vi "Uniform White Noise PtByPt.vi"(1 "initialize":bool, 2 "seed":i32=-1, 3 "amplitude":dbl=1.0 format="%0.2f") -> (0 "uniform white noise":dbl format="%0.2f")   [LabVIEW 2020, in "NI_PtbyPt.lvlib"]
doc: "Generates a uniformly distributed, pseudorandom pattern whose values are in the range [-a:a], where a is the absolute value of <B>amplitude</B>."
uses:
  NI_PtbyPt.lvlib
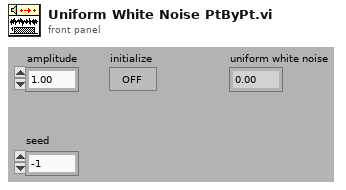
[diagram p1: front panel]
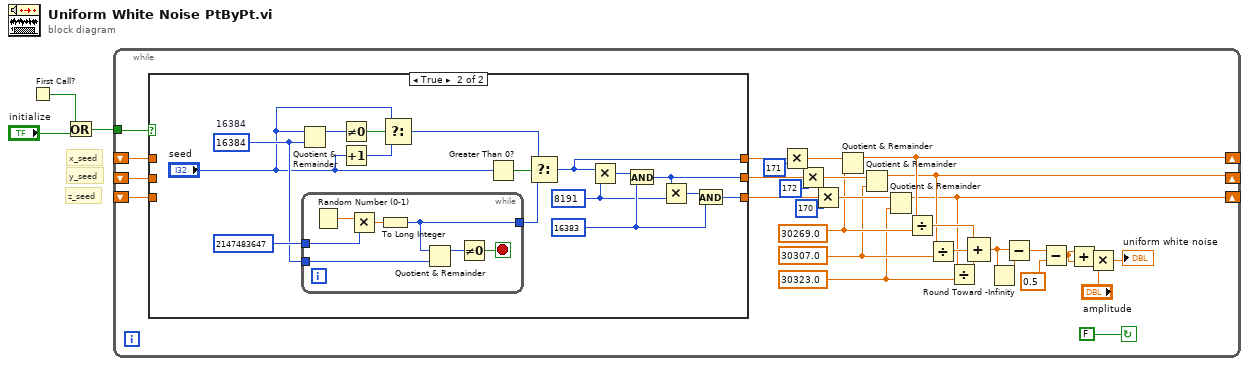
[diagram p0: block diagram]
diagram:
  # "z_seed"
  # "y_seed"
  # "x_seed"
  n1 = First Call?() -> (First Call?: T/F=w2:bool)
  n2 = Or(x=w2, y="initialize") -> (x .or. y?=w1:bool)
  n3 = while {
    tunnel: w1 -> [w10]
    shift-left: _ -> [w31]
    shift-right: [w12] -> _
    shift-left: _ -> [w32]
    shift-right: [w14] -> _
    shift-left: _ -> [w33]
    shift-right: [w16] -> _
    stop <- FALSE continue-if-true
    w11 = 30323.0
    w13 = 30307.0
    w15 = 30269.0
    n4 = case shown="True" w10 {
      tunnel: w33 -> [w37 _]
      tunnel: w32 -> [w36 _]
      tunnel: w31 -> [w35 _]
      tunnel: [w37 w38] -> w30
      tunnel: [w35 w53] -> w29
      tunnel: [w36 w52] -> w28
      frame False {
      }
      frame True {
        w46 = 16384  # 16384
        w50 = 16383
        w48 = 8191 ("y")
        n5 = Quotient & Remainder(x="seed", y=w46) -> (x-y*floor(x/y)=w41:i32)  [unwired: 1 out]
        n6 = while {
          tunnel: [w58] -> w45
          tunnel: w46 -> [w57]
          tunnel: 2147483647 ("x") -> [w54]
          stop <- w55 stop-if-true
          n7 = Random Number (0-1)() -> (number: 0 to 1=w59:dbl)
          n8 = Multiply(x=w59, y=w54) -> (x*y=w60:dbl)
          n9 = To Long Integer(number=w60) -> (32bit integer=w58:i32)
          n10 = Quotient & Remainder(x=w58, y=w57) -> (x-y*floor(x/y)=w56:i32)  [unwired: 1 out]
          n11 = Not Equal To 0?(x=w56) -> (x != 0?=w55:bool)
        }
        n12 = Not Equal To 0?(x=w41) -> (x != 0?=w42:bool)
        n13 = Increment(x="seed") -> (x+1=w43:i32)
        n14 = Select(t="seed", s=w42, f=w43) -> (s? t:f=w44:i32)
        n15 = Greater Than 0?(x="seed") -> (x > 0?=w40:bool)
        n16 = Select(t=w44, s=w40, f=w45) -> (s? t:f=w38:i32)
        n17 = Multiply(x=w38, y=w48) -> (x*y=w51:i32)
        n18 = And(x=w51, y=w50) -> (x .and. y?=w52:i32)
        n19 = Multiply(x=w52, y=w48) -> (x*y=w49:i32)
        n20 = And(x=w49, y=w50) -> (x .and. y?=w53:i32)
      }
    }
    n21 = Multiply(x=w30, y=171) -> (x*y=w17:dbl)
    n22 = Multiply(x=w28, y=172) -> (x*y=w25:dbl)
    n23 = Multiply(x=w29, y=170) -> (x*y=w24:dbl)
    n24 = Quotient & Remainder(x=w17, y=w15) -> (x-y*floor(x/y)=w16:dbl)  [unwired: 1 out]
    n25 = Quotient & Remainder(x=w25, y=w13) -> (x-y*floor(x/y)=w14:dbl)  [unwired: 1 out]
    n26 = Quotient & Remainder(x=w24, y=w11) -> (x-y*floor(x/y)=w12:dbl)  [unwired: 1 out]
    n27 = Divide(x=w16, y=w15) -> (x/y=w23:dbl)
    n28 = Divide(x=w14, y=w13) -> (x/y=w22:dbl)
    n29 = Divide(x=w12, y=w11) -> (x/y=w21:dbl)
    n30 = Compound Arithmetic op=ADD(w23, w22, w21) -> (w20:dbl)
    n31 = Round Toward -Infinity(1:w20) -> (0:w19:dbl)
    n32 = Subtract(x=w20, y=w19) -> (x-y=w7:dbl)
    n33 = Subtract(x=w7, y=0.5) -> (x-y=w4:dbl)
    n34 = Add(x=w4, y=w4) -> (x+y=w5:dbl)
    n35 = Multiply(x=w5, y="amplitude") -> (x*y=→"uniform white noise":dbl)
  }
